vi "Read.vi"(8 "error in (no error)":errorcluster, 11 "DAQ Actor in":refnum<class "DAQ Actor.lvclass">) -> (0 "error out":errorcluster, 3 "DAQ Actor out":refnum<class "DAQ Actor.lvclass">)   [LabVIEW 2017, in "DAQ Actor.lvlib" / "DAQ Actor.lvclass"]
uses:
  DAQ Actor.lvclass
  C:/Program Files (x86)/National Instruments/LabVIEW 2017/vi.lib/ActorFramework/Actor/Actor.lvclass
  <vilib>/ActorFramework/Actor/Actor.lvclass/Actor.ctl
  DAQ Actor.lvclass/DAQ Actor.ctl
  UI Actor Messages/Update Data Ind Msg/Update Data Ind Msg.lvclass/Update Data Ind Msg.ctl
  <vilib>/ActorFramework/Message Enqueuer/Message Enqueuer.lvclass/Message Enqueuer.ctl
  <vilib>/DAQmx/read.llb/DAQmx Read (Analog DBL 1Chan 1Samp).vi
  <vilib>/ActorFramework/Message Enqueuer/Enqueue.vi
  UI Actor Messages/Update Data Ind Msg/Update Data Ind Msg.lvclass
  C:/Program Files (x86)/National Instruments/LabVIEW 2017/vi.lib/ActorFramework/Message/Message.lvclass
  <vilib>/DAQmx/miscellaneous.llb/DAQmx Fill In Error Info.vi
  <vilib>/ActorFramework/Message Priority Queue/Priority Enqueue.vi
  <vilib>/ActorFramework/Actor/Actor.lvclass
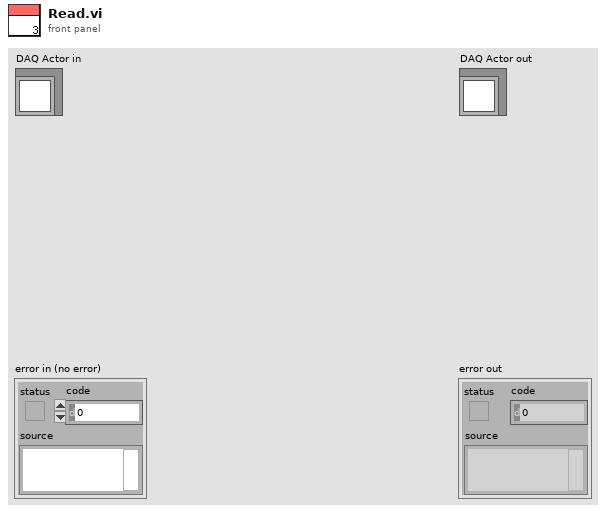
[diagram p1: front panel]
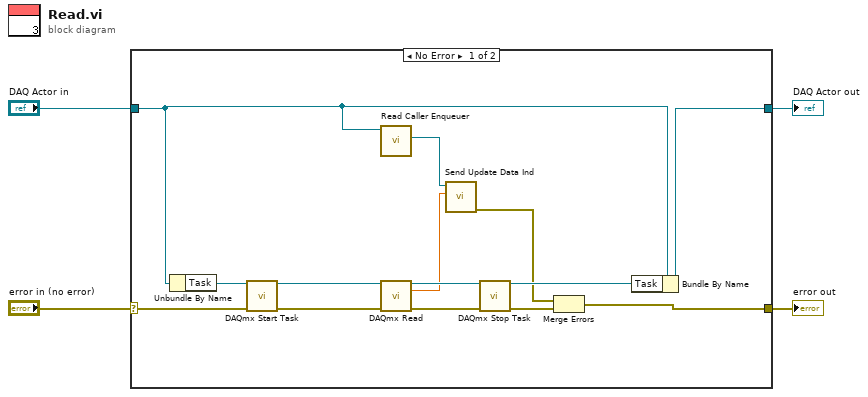
[diagram p0: block diagram]
diagram:
  n1 = case shown="No Error" "error in (no error)" {
    selector: "error in (no error)" -> [w18 w20]
    tunnel: [w7 w20] -> w3
    tunnel: [w17 w19] -> w1
    tunnel: "DAQ Actor in" -> [w5 w19]
    frame No Error {
      n2 = Unbundle By Name(w5) -> ("Task"=w13:refnum<k21>)
      n3 = call <vilib>:"DAQmx Start Task.vi"("task/channels in"=w13, "error in"=w18) -> ("task out"=w12:refnum<k21>, "error out"=w16:errorcluster)  [unwired: 12 in]
      n4 = call <vilib>:"Read Caller Enqueuer.vi"("Actor"=w5) -> ("Caller Enqueuer"=w9:refnum<class "Message Enqueuer.lvclass">)  [unwired: 10 in]
      n5 = call-poly <vilib>:"DAQmx Read.vi"("task/channels in"=w12, "error in"=w16) -> ("task out"=w11:refnum<k21>, "data"=w8:dbl, "error out"=w15:errorcluster)  [unwired: 11 in]
      n6 = call "Send Update Data Ind.vi"("Measurement"=w8, "Message Enqueuer"=w9) -> ("error out"=w6:errorcluster)  [unwired: 8 in, 1 out]
      n7 = call <vilib>:"DAQmx Stop Task.vi"("task/channels in"=w11, "error in"=w15) -> ("task out"=w10:refnum<k21>, "error out"=w14:errorcluster)  [unwired: 12 in]
      n8 = Merge Errors(w6, w14) -> (w7:errorcluster)
      n9 = Bundle By Name(cluster=w5, "Task"=w10) -> (w17:refnum<class "DAQ Actor.lvclass">)
    }
    frame Error {
    }
  }
  "error out" <- w3
  "DAQ Actor out" <- w1
